vi "Do.vi"(8 "error in":errorcluster, 10 "Actor in":refnum<class "Actor.lvclass">, 11 "Start Write PAS Wvfm MSG":refnum<class "Start Write PAS Wvfm MSG.lvclass">) -> (0 "error out":errorcluster, 2 "Actor out":refnum<class "Actor.lvclass">)   [LabVIEW 2018, in "Controller.lvlib" / "Start Write PAS Wvfm MSG.lvclass"]
doc: "(<B>Filename</B>: Actor Framework.lvlib:Message.lvclass:Do.vi)\n\nDefines what a message does when it is received by an actor. Generally, a message instructs an actor to invoke one of its methods. By default, this method does nothing. A child class must override it to define behavior."
uses:
  Start Write PAS Wvfm MSG.lvclass
  <vilib>/ActorFramework/Actor/Actor.lvclass
  Commands/Exe Write PAS Wvfm CMD/Exe Write PAS Wvfm CMD.lvclass
  G:/sw_repo/For Builds/Nicholas/File Actor/Messages/Abstract/Exe Write/Exe Write.lvclass
  File Actor/File Actor.lvclass
  C:/Program Files (x86)/National Instruments/LabVIEW 2018/vi.lib/MSR Consulting, LLC/General Reuse/SuperActor/SuperActor.lvclass
  C:/Program Files (x86)/National Instruments/LabVIEW 2018/vi.lib/ActorFramework/Actor/Actor.lvclass
  gController.lvclass
  gController.lvclass/gController.ctl
  Commands/Exe Write PAS Wvfm CMD/Exe Write PAS Wvfm CMD.lvclass/Exe Write PAS Wvfm CMD.ctl
  <vilib>/MSR Consulting, LLC/General Reuse/SuperActor/SuperActor.lvclass/SuperActor.ctl
  File Actor/File Actor.lvclass/File Actor.ctl
  Read DataMap.vi
  <vilib>/MSR Consulting, LLC/General Reuse/SuperActor/Write ID.vi
  File Actor/Write Cfg Header.vi
  File Actor/Write Exe Write.vi
  Commands/Exe Write PAS Wvfm CMD/Write DataMap.vi
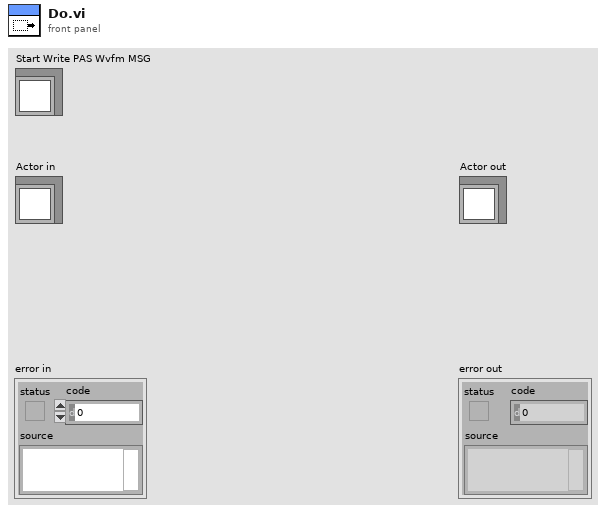
[diagram p1: front panel]
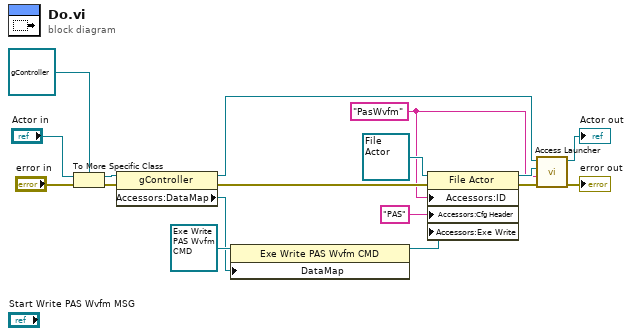
[diagram p0: block diagram]
diagram:
  w4 = "PasWvfm" ("name")
  n1 = To More Specific Class(target class=refnum<class "gController.lvclass"> refnum ("Controller.lvlib:gController"), reference="Actor in", error in="error in") -> (specific class reference=w15:refnum<class "gController.lvclass">, error out=w13:errorcluster)
  n2 = property class="gController"(reference=w15, error in=w13) -> (reference out=w6:refnum<class "gController.lvclass">, error out=w7:errorcluster, "Accessors:DataMap"=w10:refnum<data-value>)
  n3 = property class="Exe Write PAS Wvfm CMD"(reference=refnum<class "Exe Write PAS Wvfm CMD.lvclass"> refnum ("Controller.lvlib:Exe Write PAS Wvfm CMD.lvclass"), "DataMap"=w10) -> (reference out=w9:refnum<class "Exe Write PAS Wvfm CMD.lvclass">)  [unwired: 1 in, 1 out]
  n4 = property class="File Actor"(reference=refnum<class "File Actor.lvclass"> refnum ("File Library.lvlib:File Actor"), error in=w7, "Accessors:ID"=w4, "Accessors:Cfg Header"="PAS" ("Cfg Header"), "Accessors:Exe Write"=w9) -> (reference out=w5:refnum<class "File Actor.lvclass">, error out=w2:errorcluster)
  n5 = call "Access Launcher.vi"("error in (no error)"=w2, "ID"=w4, "Nested Actor"=w5, "gController in"=w6) -> ("error out"=→"error out":errorcluster, "gController out"=→"Actor out":refnum<class "gController.lvclass">)  [unwired: 5 in, 1 out]
